vi "DCAM_daq_example_acquire_both.vi"() -> ()   [LabVIEW 2015]
uses:
  <vilib>/DAQmx/read.llb/DAQmx Read (Digital 1D Wfm NChan NSamp).vi
  <vilib>/DAQmx/read.llb/DAQmx Read (Analog 1D Wfm NChan NSamp).vi
  <vilib>/DAQmx/create/channels.llb/DAQmx Create Channel (AI-Voltage-Basic).vi
  <vilib>/DAQmx/configure/timing.llb/DAQmx Timing (Sample Clock).vi
  <vilib>/DAQmx/create/channels.llb/DAQmx Create Channel (DI-Digital Input).vi
  <vilib>/DAQmx/miscellaneous.llb/DAQmx Fill In Error Info.vi
  <resource>/objmgr/daqmx.rc
panel:
  out "x != 0?":bool
  out "error out":errorcluster
  out "DCAM Ver.":string
  out "Library Ver.":string
  out "Firmware":string
  out "Camera ID":string
  out "Model":string
  out "Timeseries Base Filename":string
  out "Timeseries save path":path
  in  "Start Button":bool
  out "Image":u16[][](graph)
  in  "stop":bool
  out "Frames Recorded":i32
  in  "Frames":i32=100
  out "Waveform Chart 2":waveform(dbl)[](graph)
  out "Actual Sample Rate Dev1 DIO":dbl=1000.0 format="%0.2f"
  out "Actual Sample Rate Dev2":dbl=1000.0 format="%0.2f"
  out "Waveform Chart":waveform(dbl)[](graph)
  out "Actual Sample Rate Dev1":dbl=1000.0 format="%0.2f"
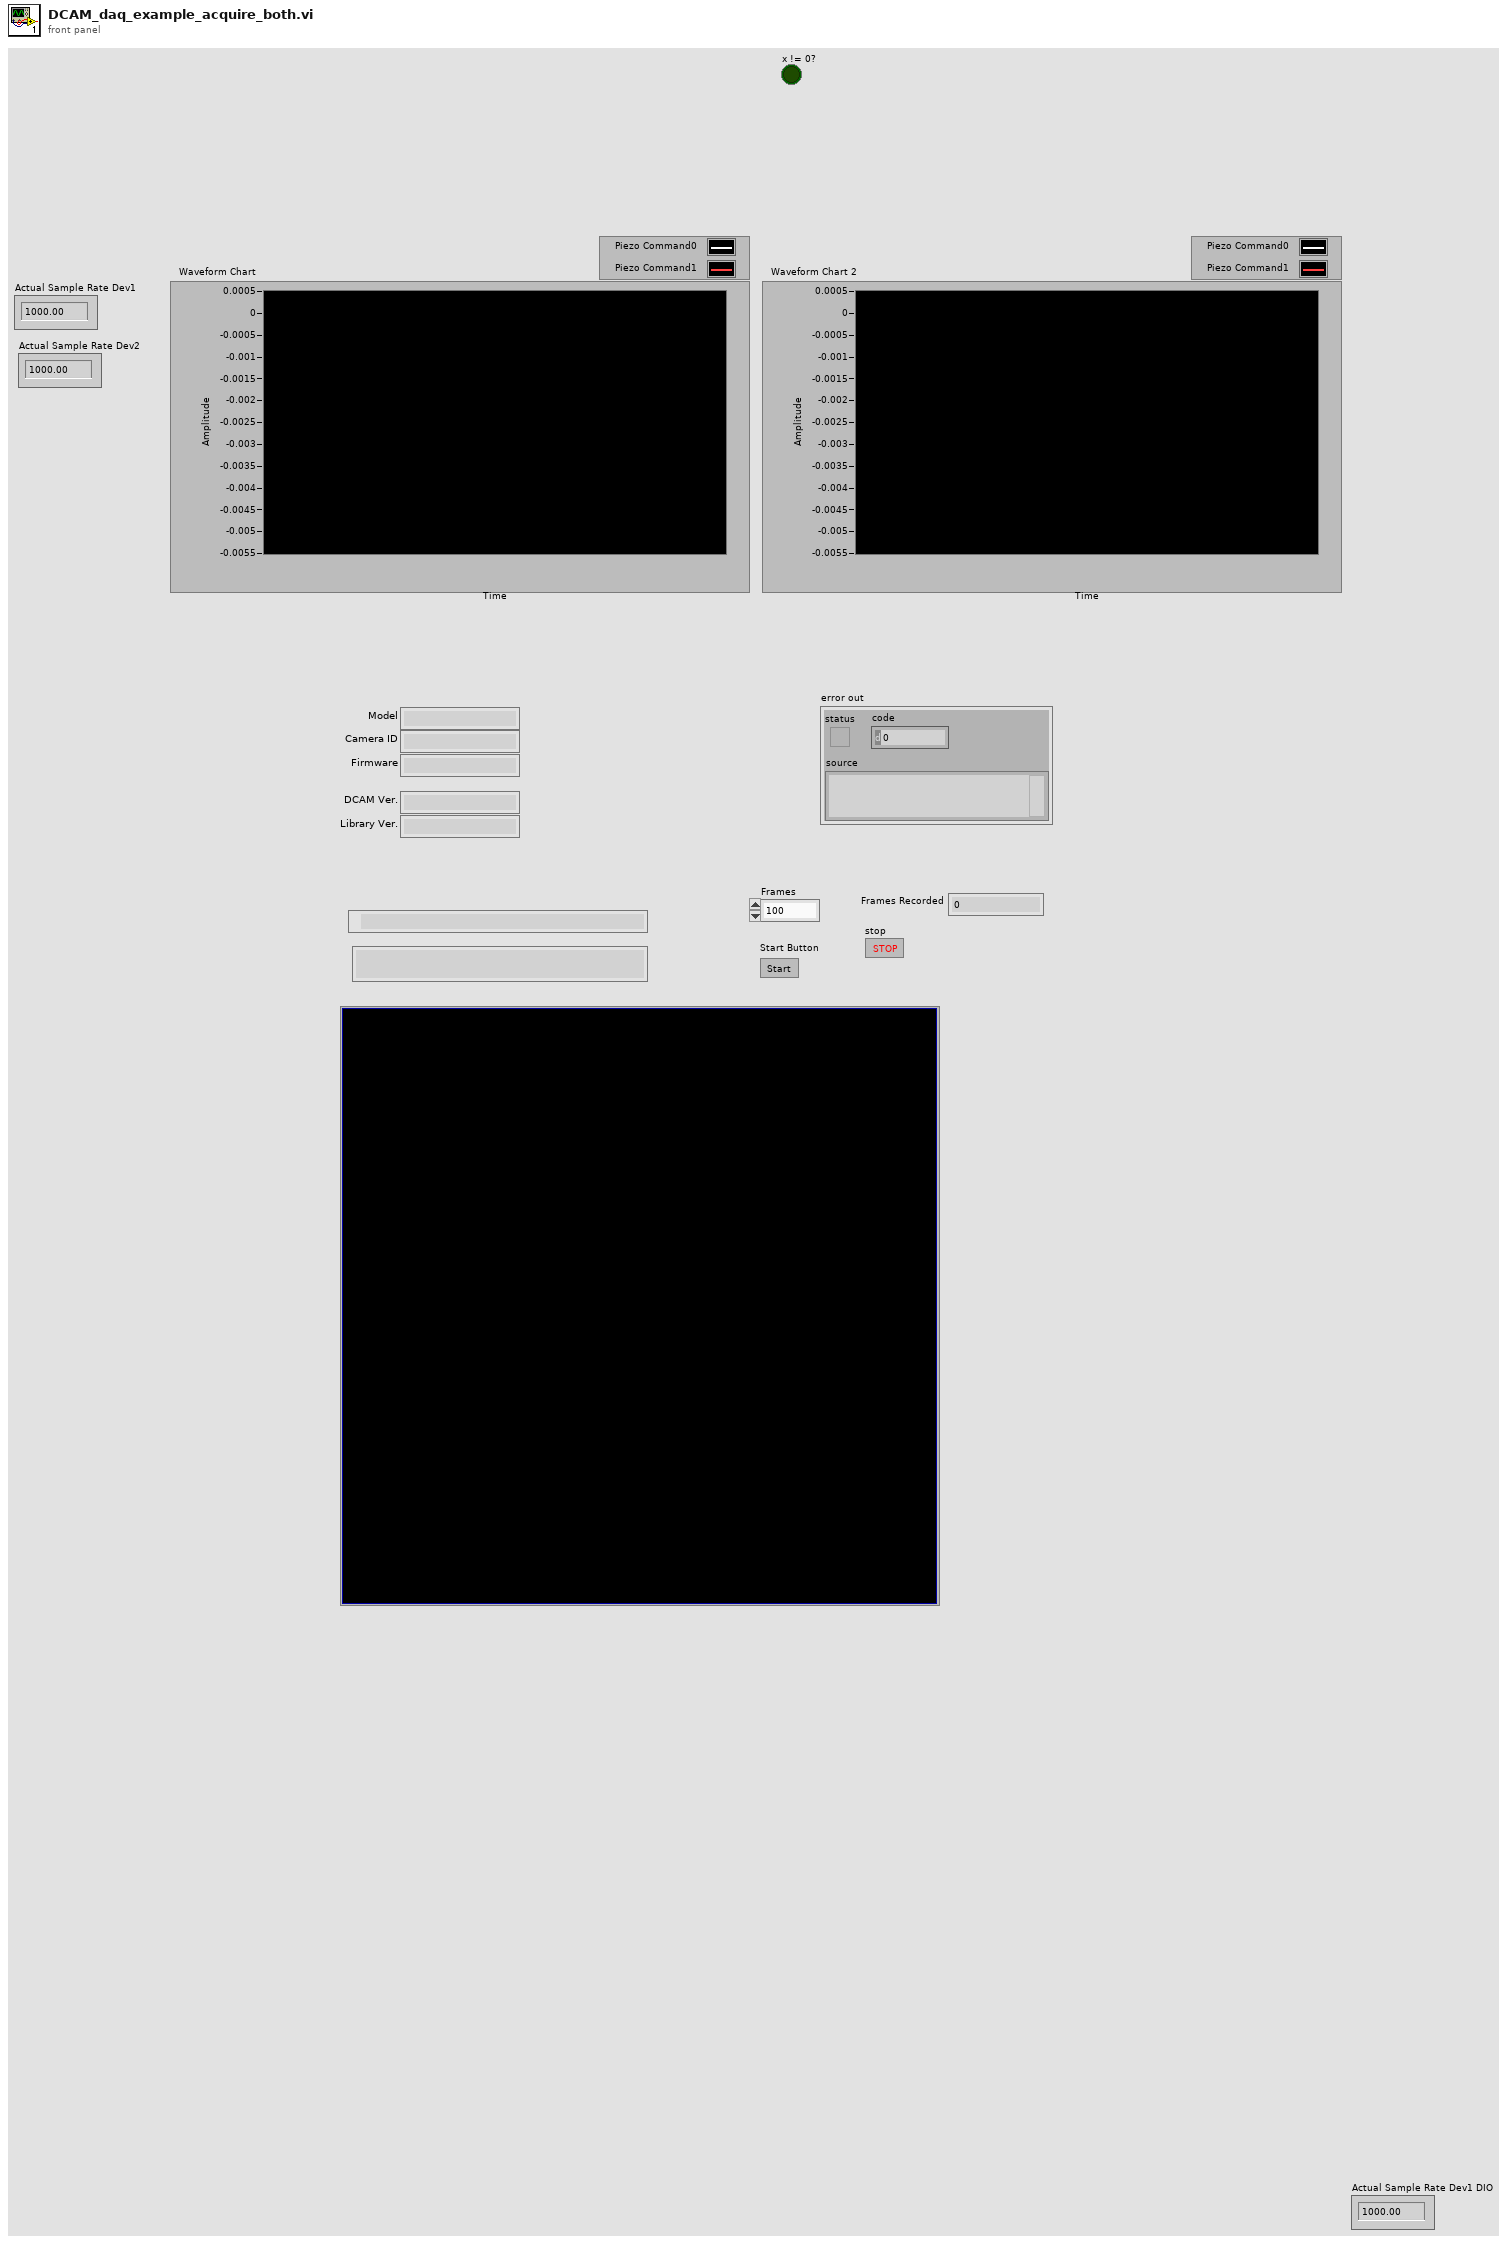
[diagram p1: front panel]
types:
  T1 = cluster{"Capture Library":string, "DCAM-API":string}
  T2 = cluster{"Model":string, "Camera ID":string, "Firmware":string}
  T3 = cluster{"height":u32, "width":u32, "datatype":u32}
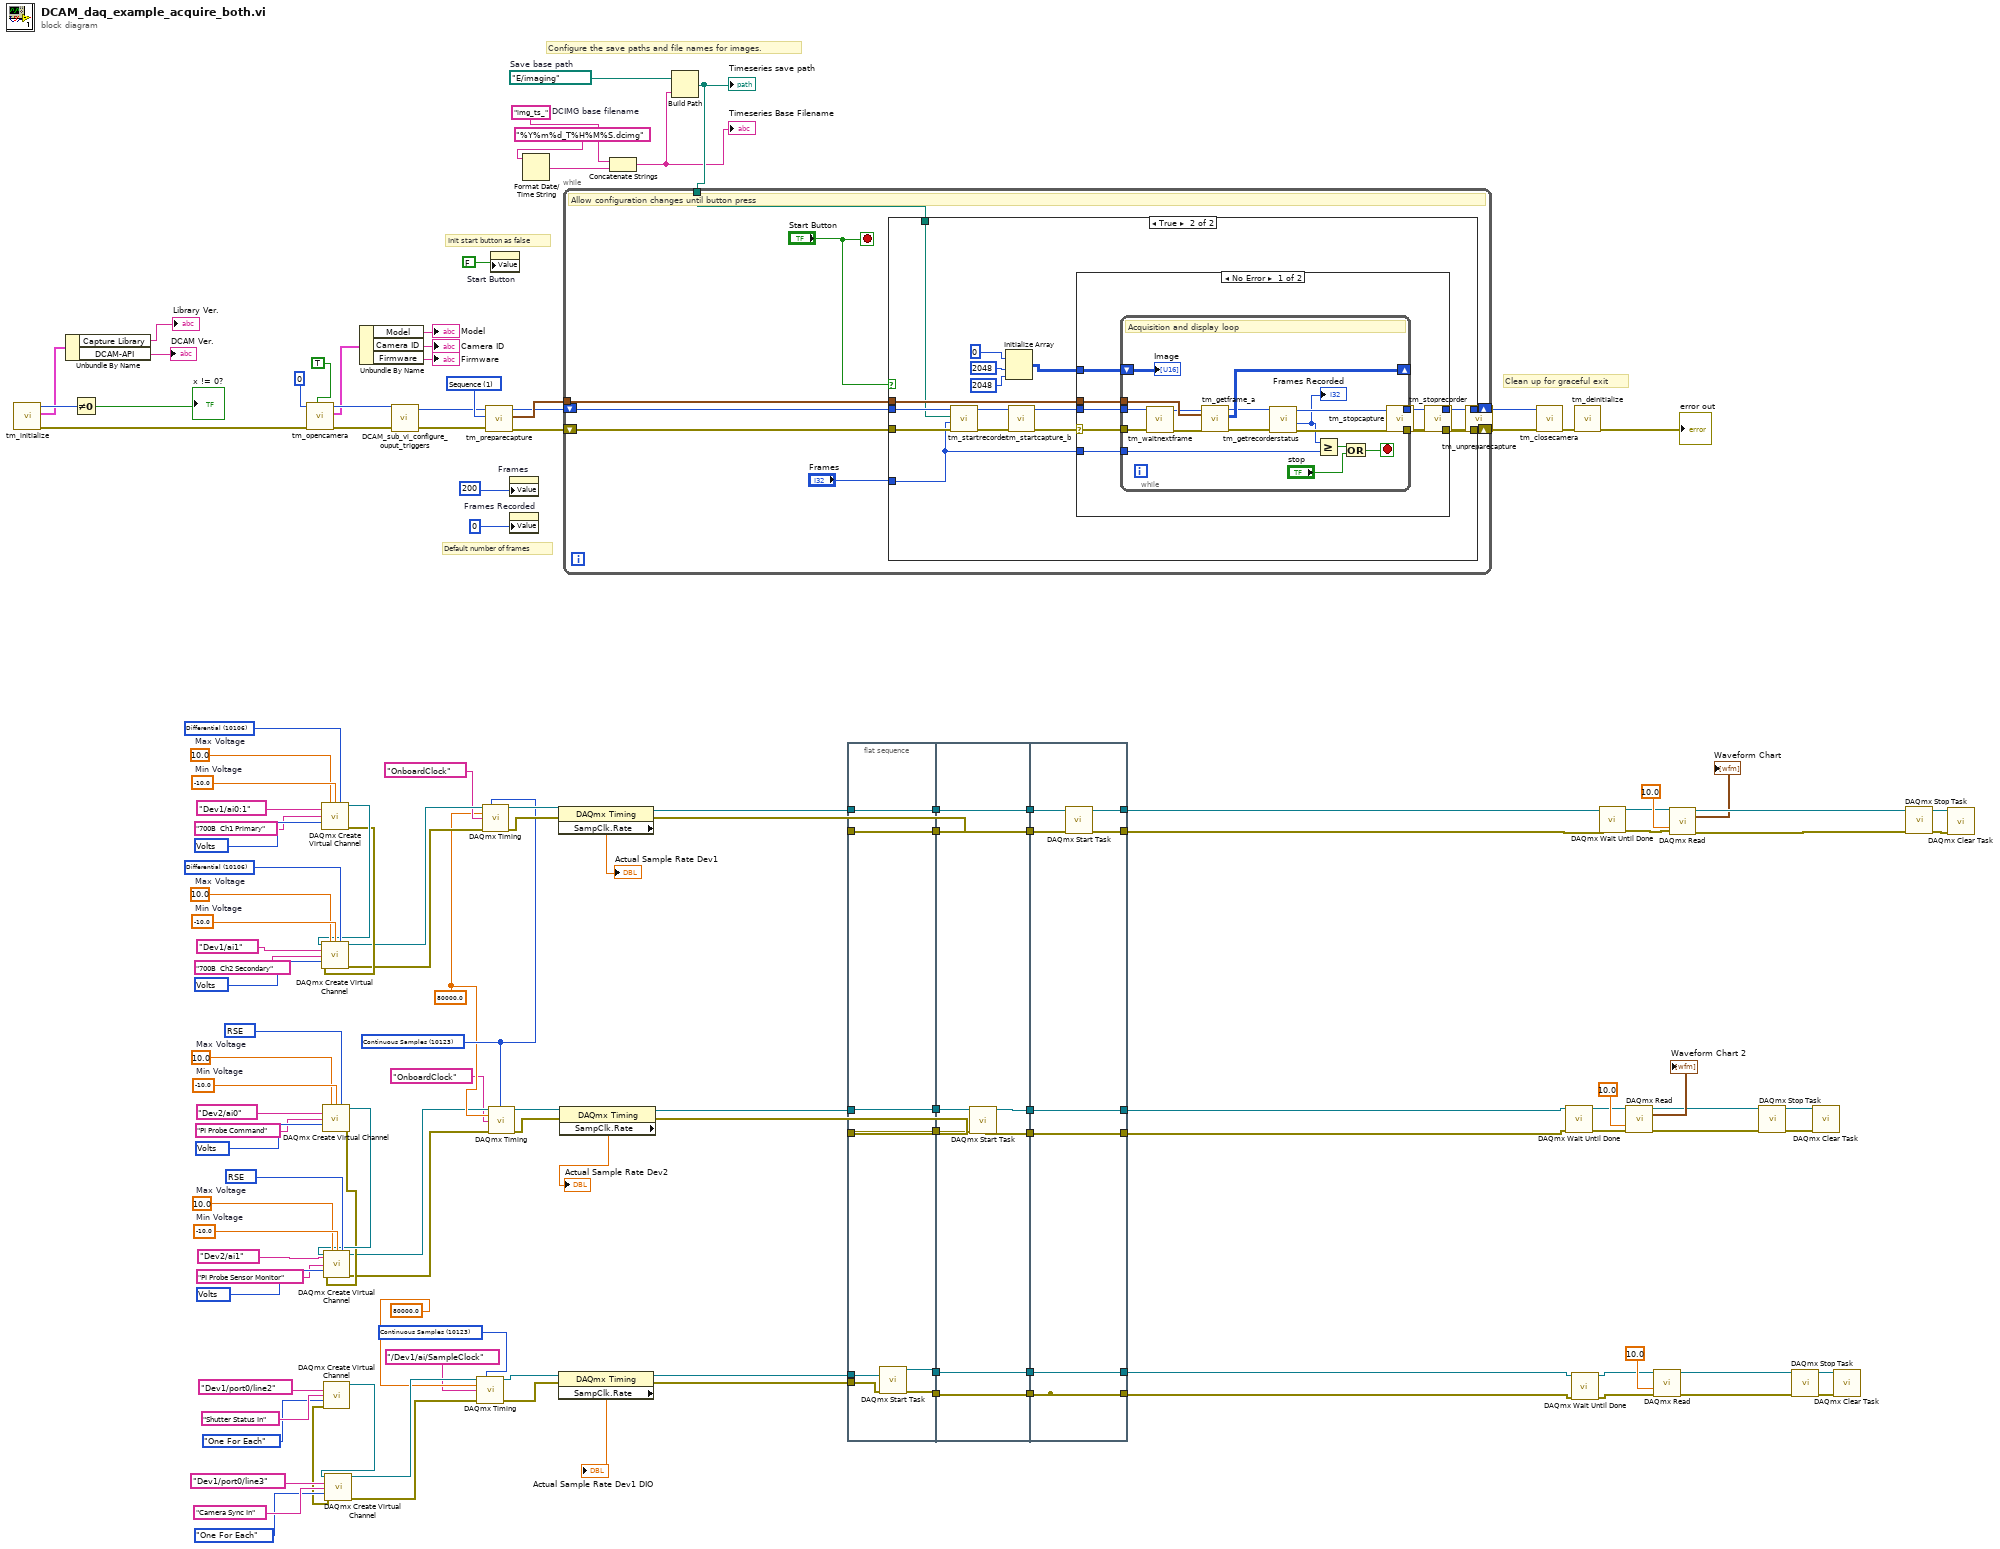
[diagram p0: block diagram]
diagram:
  w21 = 1 items=["Snap", "Sequence"] ("Capture mode")
  w5 = "img_ts_"  # DCIMG base filename
  w8 = path "E:/imaging"  # Save base path
  w76 = 10123 items=["Finite Samples"=10178, "Continuous Samples"=10123] ("sample mode")
  w109 = 10348 items=["Volts"=10348, "From Custom Scale"=10065] ("units")
  w110 = 10083 items=["default"=-1, "RSE"=10083, "NRSE"=10078, "Differential"=10106, "Pseudodifferential"=12529] ("input terminal configuration")
  w112 = -10.0  # Min Voltage
  w111 = 10.0  # Max Voltage
  w114 = 10348 items=["Volts"=10348, "From Custom Scale"=10065] ("units")
  w115 = 10083 items=["default"=-1, "RSE"=10083, "NRSE"=10078, "Differential"=10106, "Pseudodifferential"=12529] ("input terminal configuration")
  w117 = -10.0  # Min Voltage
  w116 = 10.0  # Max Voltage
  w103 = 10123 items=["Finite Samples"=10178, "Continuous Samples"=10123] ("sample mode")
  w101 = 80000.0
  w137 = 10348 items=["Volts"=10348, "From Custom Scale"=10065] ("units")
  w138 = 10106 items=["default"=-1, "RSE"=10083, "NRSE"=10078, "Differential"=10106, "Pseudodifferential"=12529] ("input terminal configuration")
  w140 = -10.0  # Min Voltage
  w139 = 10.0  # Max Voltage
  w141 = 10348 items=["Volts"=10348, "From Custom Scale"=10065] ("units")
  w142 = 10106 items=["default"=-1, "RSE"=10083, "NRSE"=10078, "Differential"=10106, "Pseudodifferential"=12529] ("input terminal configuration")
  w144 = -10.0  # Min Voltage
  w143 = 10.0  # Max Voltage
  # "Init start button as false"
  # "Clean up for graceful exit"
  # "Default number of frames"
  # "Configure the save paths and file names for images."
  n1 = call <userlib>:"tm_initialize.vi"() -> ("error out"=w34:errorcluster, "Version Info"=w37:T1, "Number Of Cameras"=w39:u32)  [unwired: 8 in, 1 out]
  n2 = Unbundle By Name(w37) -> ("Capture Library"=→"Library Ver.":string, "DCAM-API"=→"DCAM Ver.":string)
  n3 = Not Equal To 0?(x=w39) -> (x != 0?=→"x != 0?":bool)
  n4 = call <userlib>:"tm_opencamera.vi"("Force Open"=TRUE, "error in (no error)"=w34, "Camera Index"=0) -> ("error out"=w29:errorcluster, "Camera Details"=w25:T2, "Handle out"=w30:u32)  [unwired: 6 in]
  n5 = call-poly <vilib>:"DAQmx Create Virtual Channel.vi"("maximum value"=w143, "minimum value"=w144, "input terminal configuration"=w142, "physical channels"=tag "Dev1/ai0:1" ("DAQmx Physical Channel"), "name to assign"="700B  Ch1 Primary", "units"=w141) -> ("task out"=w135:refnum<k21>, "error out"=w134:errorcluster)  [unwired: 8 in]
  n6 = call-poly <vilib>:"DAQmx Create Virtual Channel.vi"("task in"=w135, "maximum value"=w139, "minimum value"=w140, "input terminal configuration"=w138, "physical channels"=tag "Dev1/ai1" ("DAQmx Physical Channel"), "name to assign"="700B  Ch2 Secondary", "units"=w137, "error in"=w134) -> ("task out"=w119:refnum<k21>, "error out"=w118:errorcluster)  [unwired: 6 in]
  n7 = call-poly <vilib>:"DAQmx Create Virtual Channel.vi"("maximum value"=w116, "minimum value"=w117, "input terminal configuration"=w115, "physical channels"=tag "Dev2/ai0" ("DAQmx Physical Channel"), "name to assign"="PI Probe Command", "units"=w114) -> ("task out"=w107:refnum<k21>, "error out"=w106:errorcluster)  [unwired: 8 in]
  n8 = call-poly <vilib>:"DAQmx Create Virtual Channel.vi"("task in"=w107, "maximum value"=w111, "minimum value"=w112, "input terminal configuration"=w110, "physical channels"=tag "Dev2/ai1" ("DAQmx Physical Channel"), "name to assign"="PI Probe Sensor Monitor", "units"=w109, "error in"=w106) -> ("task out"=w100:refnum<k21>, "error out"=w99:errorcluster)  [unwired: 6 in]
  n9 = call-poly <vilib>:"DAQmx Create Virtual Channel.vi"("lines"=tag "Dev1/port0/line2" ("DAQmx Physical Channel"), "name to assign"="Shutter Status In", "line grouping"=enum16{"One For Each", "One For All"}."One For Each") -> ("task out"=w81:refnum<k21>, "error out"=w80:errorcluster)  [unwired: 11 in]
  n10 = call-poly <vilib>:"DAQmx Create Virtual Channel.vi"("task in"=w81, "lines"=tag "Dev1/port0/line3" ("DAQmx Physical Channel"), "name to assign"="Camera Sync In", "line grouping"=enum16{"One For Each", "One For All"}."One For Each", "error in"=w80) -> ("task out"=w78:refnum<k21>, "error out"=w79:errorcluster)  [unwired: 9 in]
  n11 = Unbundle By Name(w25) -> ("Model"=→"Model":string, "Camera ID"=→"Camera ID":string, "Firmware"=→"Firmware":string)
  n12 = call "DCAM_sub_vi_configure_ouput_triggers.vi"("error in (no error)"=w29, "Handle in"=w30) -> ("error out"=w20:errorcluster, "Handle out"=w19:u32)  [unwired: 2 in]
  n13 = call-poly <vilib>:"DAQmx Timing.vi"("task/channels in"=w78, "sample mode"=w76, "rate"=80000.0, "source"=tag "/Dev1/ai/SampleClock" ("Sample Clock Source"), "error in"=w79) -> ("task out"=w89:refnum<k21>, "error out"=w88:errorcluster)  [unwired: 9 in]
  n14 = call-poly <vilib>:"DAQmx Timing.vi"("task/channels in"=w119, "sample mode"=w103, "rate"=w101, "source"=tag "OnboardClock" ("Sample Clock Source"), "error in"=w118) -> ("task out"=w133:refnum<k21>, "error out"=w132:errorcluster)  [unwired: 9 in]
  n15 = call <userlib>:"tm_preparecapture.vi"("error in (no error)"=w20, "Capture mode"=w21, "Handle in"=w19) -> ("error out"=w16:errorcluster, "Buffer Info"=w18:T3, "Handle out"=w17:u32)  [unwired: 5 in, 1 out]
  n16 = call-poly <vilib>:"DAQmx Timing.vi"("task/channels in"=w100, "sample mode"=w103, "rate"=w101, "source"=tag "OnboardClock" ("Sample Clock Source"), "error in"=w99) -> ("task out"=w97:refnum<k21>, "error out"=w96:errorcluster)  [unwired: 9 in]
  n17 = property on="Start Button" class="Bool (strict)"("Value"=FALSE) -> ()  [unwired: 2 in, 2 out]
  n18 = property on="Frames" class="DigNum (strict)"("Value"=200) -> ()  [unwired: 2 in, 2 out]
  n19 = property on="Frames Recorded" class="DigNum (strict)"("Value"=0) -> ()  [unwired: 2 in, 2 out]
  n20 = Format Date/Time String(time format string (%c)="%Y%m%d_T%H%M%S.dcimg" ("name or relative path")) -> (date/time string=w6:string)  [unwired: 2 in]
  n21 = property class="DAQmx Timing"(reference=w133, error in=w132) -> (reference out=w131:refnum<k21>, error out=w130:errorcluster, "SampClk.Rate"=→"Actual Sample Rate Dev1":dbl)
  n22 = property class="DAQmx Timing"(reference=w89, error in=w88) -> (reference out=w91:refnum<k21>, error out=w90:errorcluster, "SampClk.Rate"=→"Actual Sample Rate Dev1 DIO":dbl)
  n23 = property class="DAQmx Timing"(reference=w97, error in=w96) -> (reference out=w94:refnum<k21>, error out=w93:errorcluster, "SampClk.Rate"=→"Actual Sample Rate Dev2":dbl)
  n24 = Concatenate Strings(w5, w6) -> (w3:string)
  "Timeseries Base Filename" <- w3
  n25 = Build Path(base path=w8, name or relative path=w3) -> (appended path=w4:path)
  "Timeseries save path" <- w4
  n26 = while {
    tunnel: w18 -> [w152]
    tunnel: w4 -> [w147]
    shift-right: [w149] -> w14
    shift-left: w17 -> [w151]
    shift-right: [w148] -> w13
    shift-left: w16 -> [w150]
    stop <- "Start Button" stop-if-true
    # "Allow configuration changes until button press"
    n27 = case shown="True" "Start Button" {
      tunnel: w152 -> [_ w169]
      tunnel: w151 -> [w154 w161]
      tunnel: w150 -> [w153 w160]
      tunnel: [w154 w159] -> w149
      tunnel: [w153 w158] -> w148
      tunnel: "Frames" -> [_ w157]
      tunnel: w147 -> [_ w155]
      frame False {
      }
      frame True {
        n28 = call <userlib>:"tm_startrecorder.vi"("error in (no error)"=w160, "frames"=w157, "File"=w155, "Handle in"=w161) -> ("error out"=w163:errorcluster, "Handle out"=w162:u32)  [unwired: 6 in]
        n29 = Initialize Array(u16 0 ("element"), 2048 ("dimension size"), 2048 ("dimension size")) -> (w164:u16[][])
        n30 = call <userlib>:"tm_startcapture_b.vi"("error in (no error)"=w163, "Handle in"=w162) -> ("error out"=w156:errorcluster, "Handle out"=w168:u32)  [unwired: 8 in]
        n31 = case shown="No Error" w156 {
          selector: w156 -> [w170 w194]
          tunnel: w169 -> [w176 _]
          tunnel: w168 -> [w175 w193]
          tunnel: w164 -> [w174 _]
          tunnel: [w173 w193] -> w159
          tunnel: [w172 w194] -> w158
          tunnel: w157 -> [w171 _]
          frame No Error {
            n32 = while {
              tunnel: w176 -> [w192]
              tunnel: w175 -> [w191]
              tunnel: w170 -> [w188]
              shift-right: [w186] -> _
              shift-left: w174 -> [w187]
              tunnel: [w183] -> w173
              tunnel: [w182] -> w172
              tunnel: w171 -> [w177]
              stop <- w180 stop-if-true
              # "Acquisition and display loop"
              n33 = call <userlib>:"tm_waitnextframe.vi"("error in (no error)"=w188, "Handle in"=w191) -> ("error out"=w189:errorcluster, "Handle out"=w190:u32)  [unwired: 6 in, 2 out]
              n34 = call <userlib>:"tm_getframe_a.vi"("error in (no error)"=w189, "Buffer Info"=w192, "Handle in"=w190) -> ("error out"=w185:errorcluster, "Data 16"=w186:u16[][], "Handle out"=w184:u32)  [unwired: 4 in, 2 out]
              n35 = call <userlib>:"tm_getrecorderstatus.vi"("error in (no error)"=w185, "Handle"=w184) -> ("error out"=w182:errorcluster, "Count"=w178:i32, "Handle"=w183:u32)  [unwired: 6 in, 1 out]
              "Frames Recorded" <- w178
              n36 = Greater Or Equal?(x=w178, y=w177) -> (x >= y?=w179:bool)
              n37 = Or(x=w179, y="stop") -> (x .or. y?=w180:bool)
              "Image" <- w187
            }
          }
          frame Error {
          }
        }
      }
    }
  }
  n38 = flat-sequence {
    tunnel: w131 -> [w202]
    tunnel: w130 -> [w201]
    tunnel: w94 -> [w196]
    tunnel: w93 -> [w195]
    tunnel: [w202] -> w74
    tunnel: [w201] -> w72
    tunnel: w91 -> [w200]
    tunnel: w90 -> [w199]
    tunnel: [w198] -> w70
    tunnel: [w197] -> w68
    tunnel: [w196] -> w66
    tunnel: [w195] -> w65
    tunnel: w74 -> [w210]
    tunnel: [w210] -> w73
    tunnel: w72 -> [w209]
    tunnel: [w209] -> w71
    tunnel: w70 -> [w208]
    tunnel: [w208] -> w69
    tunnel: w68 -> [w207]
    tunnel: [w207] -> w67
    tunnel: w66 -> [w206]
    tunnel: w65 -> [w205]
    tunnel: [w204] -> w64
    tunnel: [w203] -> w63
    tunnel: [w217] -> w123
    tunnel: [w216] -> w124
    tunnel: [w218] -> w47
    tunnel: w73 -> [w215]
    tunnel: w71 -> [w214]
    tunnel: w69 -> [w212]
    tunnel: w67 -> [w211]
    tunnel: [w211] -> _
    tunnel: w64 -> [w218]
    tunnel: w63 -> [w213]
    tunnel: [w213] -> w46
    tunnel: [w212] -> w43
    tunnel: [w211] -> w42
    frame #0 {
      n39 = call <vilib>:"DAQmx Start Task.vi"("task/channels in"=w200, "error in"=w199) -> ("task out"=w198:refnum<k21>, "error out"=w197:errorcluster)  [unwired: 12 in]
    }
    frame #1 {
      n40 = call <vilib>:"DAQmx Start Task.vi"("task/channels in"=w206, "error in"=w205) -> ("task out"=w204:refnum<k21>, "error out"=w203:errorcluster)  [unwired: 12 in]
    }
    frame #2 {
      n41 = call <vilib>:"DAQmx Start Task.vi"("task/channels in"=w215, "error in"=w214) -> ("task out"=w216:refnum<k21>, "error out"=w217:errorcluster)  [unwired: 12 in]
    }
  }
  n42 = call <userlib>:"tm_stopcapture.vi"("error in (no error)"=w13, "Handle in"=w14) -> ("error out"=w9:errorcluster, "Handle out"=w10:u32)  [unwired: 8 in]
  n43 = call <userlib>:"tm_stoprecorder.vi"("error in (no error)"=w9, "Handle in"=w10) -> ("error out"=w11:errorcluster, "Handle out"=w12:u32)  [unwired: 8 in]
  n44 = call <userlib>:"tm_unpreparecapture.vi"("error in (no error)"=w11, "Handle in"=w12) -> ("error out"=w24:errorcluster, "Handle out"=w23:u32)  [unwired: 8 in]
  n45 = call <userlib>:"tm_closecamera.vi"("error in (no error)"=w24, "Handle in"=w23) -> ("error out"=w22:errorcluster)  [unwired: 9 in]
  n46 = call <vilib>:"DAQmx Wait Until Done.vi"("task/channels in"=w47, "error in"=w46) -> ("task out"=w44:refnum<k21>, "error out"=w45:errorcluster)  [unwired: 12 in]
  n47 = call <vilib>:"DAQmx Wait Until Done.vi"("task/channels in"=w43, "error in"=w42) -> ("task out"=w41:refnum<k21>, "error out"=w40:errorcluster)  [unwired: 12 in]
  n48 = call <userlib>:"tm_deinitialize.vi"("error in (no error)"=w22) -> ("error out"=→"error out":errorcluster)  [unwired: 10 in]
  n49 = call <vilib>:"DAQmx Wait Until Done.vi"("task/channels in"=w124, "error in"=w123) -> ("task out"=w48:refnum<k21>, "error out"=w49:errorcluster)  [unwired: 12 in]
  n50 = call-poly <vilib>:"DAQmx Read.vi"("task/channels in"=w44, "timeout"=10.0, "error in"=w45) -> ("task out"=w55:refnum<k21>, "data"=→"Waveform Chart 2":waveform(dbl)[], "error out"=w54:errorcluster)  [unwired: 10 in]
  n51 = call-poly <vilib>:"DAQmx Read.vi"("task/channels in"=w41, "timeout"=10.0, "error in"=w40) -> ("task out"=w53:refnum<k21>, "error out"=w52:errorcluster)  [unwired: 10 in, 1 out]
  n52 = call-poly <vilib>:"DAQmx Read.vi"("task/channels in"=w48, "timeout"=10.0, "error in"=w49) -> ("task out"=w127:refnum<k21>, "data"=→"Waveform Chart":waveform(dbl)[], "error out"=w126:errorcluster)  [unwired: 10 in]
  n53 = call <vilib>:"DAQmx Stop Task.vi"("task/channels in"=w55, "error in"=w54) -> ("task out"=w59:refnum<k21>, "error out"=w58:errorcluster)  [unwired: 12 in]
  n54 = call <vilib>:"DAQmx Stop Task.vi"("task/channels in"=w53, "error in"=w52) -> ("task out"=w57:refnum<k21>, "error out"=w56:errorcluster)  [unwired: 12 in]
  n55 = call <vilib>:"DAQmx Clear Task.vi"("task in"=w59, "error in"=w58) -> ()  [unwired: 13 in, 1 out]
  n56 = call <vilib>:"DAQmx Clear Task.vi"("task in"=w57, "error in"=w56) -> ()  [unwired: 13 in, 1 out]
  n57 = call <vilib>:"DAQmx Stop Task.vi"("task/channels in"=w127, "error in"=w126) -> ("task out"=w128:refnum<k21>, "error out"=w125:errorcluster)  [unwired: 12 in]
  n58 = call <vilib>:"DAQmx Clear Task.vi"("task in"=w128, "error in"=w125) -> ()  [unwired: 13 in, 1 out]
